vi "Reset VI Front Panel.vi"(8 "error in":errorcluster) -> (0 "error out":errorcluster)   [LabVIEW 2024, in "User Interface Control.lvlib"]
uses:
  User Interface Control.lvlib
  Tester Internal Communication/References - Get.vi
  Tester Internal Communication/Tester InterComm.lvlib
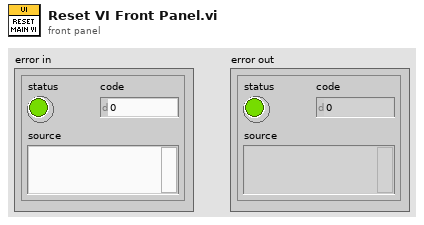
[diagram p1: front panel]
types:
  T1 = typedef "Tester InterComm.lvlib/Tester References.ctl" = cluster{"Main VI":cluster{"This VI":refnum<vi>}, "App Controls":cluster{"Test Device":refnum<vi>, "Tab Control":refnum<vi>, "STOP":refnum<vi>, "Working Mode":refnum<vi>}, "Indicators":cluster{"Messages Display":refnum<vi>, "Voltage Value":refnum<vi>, "PWM Value":refnum<vi>, "PWM Graph":refnum<vi>, "Duty Cycle":refnum<vi>, "Frequency":refnum<vi>, "Sinewave Graph":refnum<vi>, "ECU Present":refnum<vi>}, "Manufacturing Mode Controls":cluster{"Read Speed":refnum<vi>, "Voltage Out":refnum<vi>, "V Enable/Disable":refnum<vi>, "PWM Enable/Disable":refnum<vi>, "PWM Out":refnum<vi>, "Sine Enable/Disable":refnum<vi>, "Sinewave Out":refnum<vi>, "DO1":refnum<vi>, "DO2":refnum<vi>}}
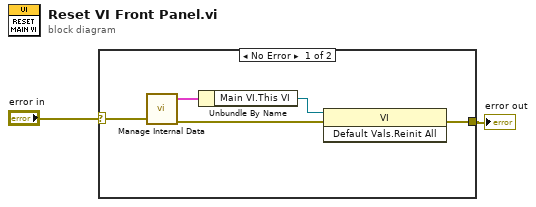
[diagram p0: block diagram]
diagram:
  n1 = case shown="No Error" "error in" {
    selector: "error in" -> [w3 w8]
    tunnel: [w4 w8] -> w2
    frame No Error {
      n2 = call-poly "Manage Internal Data.vi"("error in"=w3) -> ("error out"=w5:errorcluster, "References Out"=w7:T1)  [unwired: 9 in]
      n3 = Unbundle By Name(w7) -> ("Main VI.This VI"=w6:refnum<vi>)
      n4 = invoke class="VI" method="Default Vals.Reinit All"(reference=w6, error in=w5) -> (error out=w4:errorcluster)  [unwired: 1 in, 2 out]
    }
    frame Error {
    }
  }
  "error out" <- w2
